vi "Ball Launcher Main.vi"() -> (4 "Elapsed Time":dbl, 15 "Error Out":errorcluster)   [LabVIEW 2023, in "Ball Launcher.lvlib"]
doc: "Sampe CLD Template"
uses:
  Ball Launcher.lvlib
  Typedefs/Queue Operations.ctl
  Typedefs/Data Cluster.ctl
  Typedefs/Timer Details.ctl
  <vilib>/Utility/error.llb/Trim Whitespace One-Sided.vi
panel:
  out "Ready":bool
  in  "Launch":bool
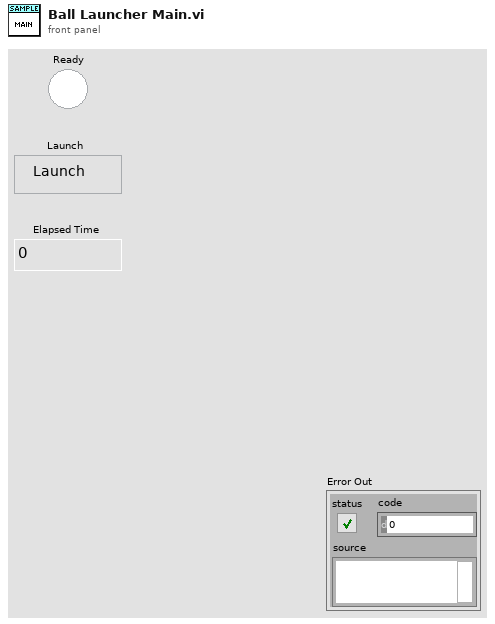
[diagram p1: front panel]
types:
  T1 = typedef "Ball Launcher.lvlib/Data Cluster.ctl" = cluster{"Timer Details":T2, "Enable Controls ref":refnum<vi>[], "Disable Controls ref":refnum<vi>[], "File Path":path, "Ready":bool}
  T2 = typedef "Ball Launcher.lvlib/Timer Details.ctl" = cluster{"Elapsed Time":dbl, "Previous Time":timestamp, "Started?":bool, "Set Time":dbl}
  T3 = typedef "Ball Launcher.lvlib/Queue Operations.ctl" = enum16{"Create Q", "Enqueue", "Enstack", "Dequeue", "Flush Q", "Release Q"}
  T4 = enum8{"Enabled", "Disabled", "Disabled and Grayed Out"}
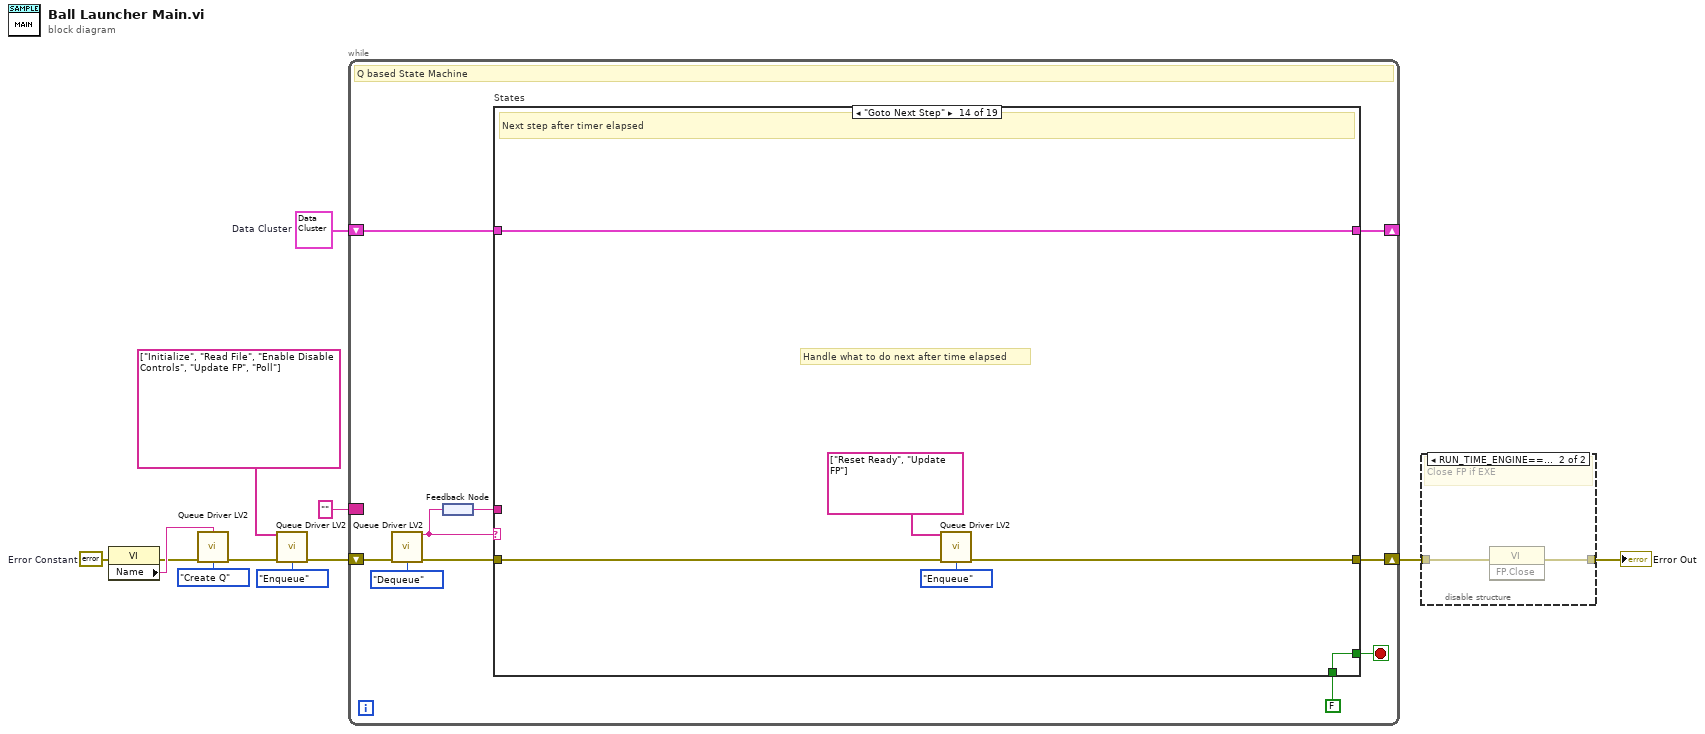
[diagram p0: block diagram]
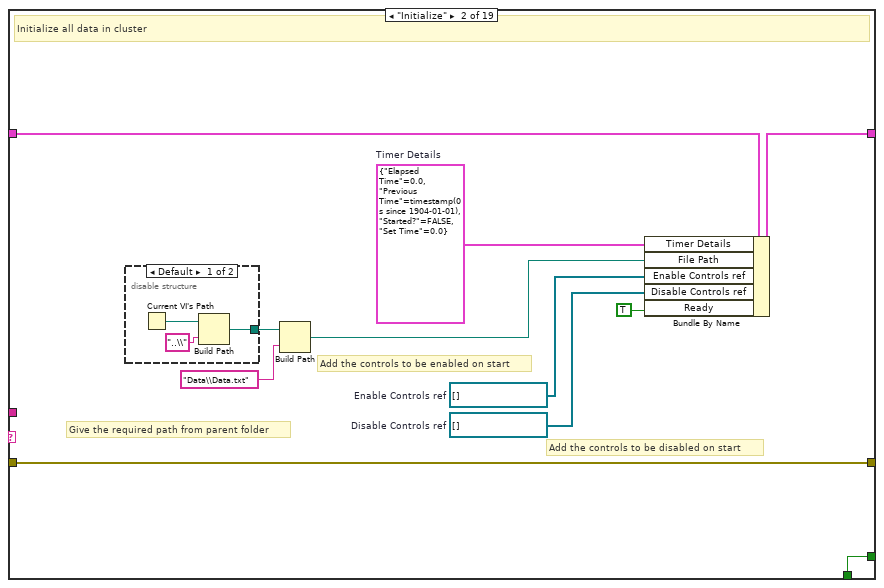
[diagram p4: hidden frame]
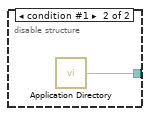
[diagram p5: hidden frame]
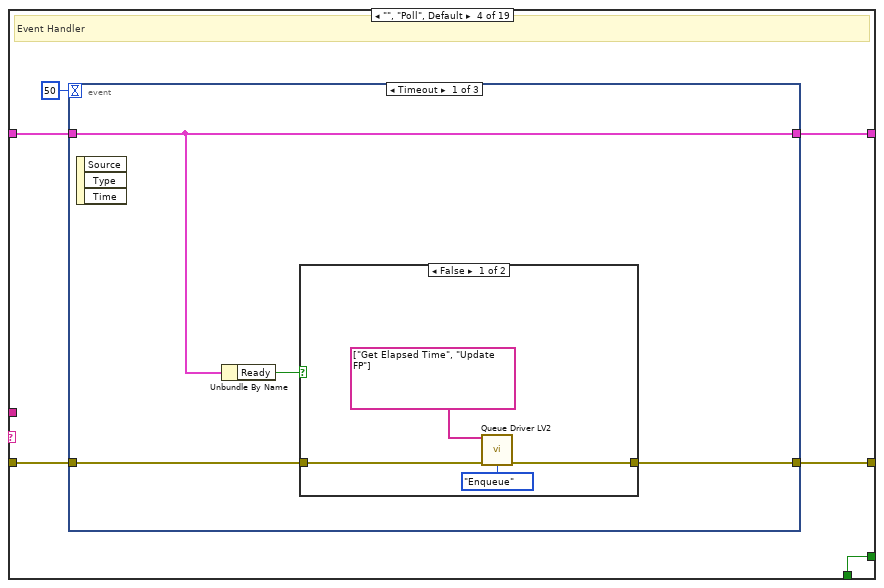
[diagram p7: hidden frame]
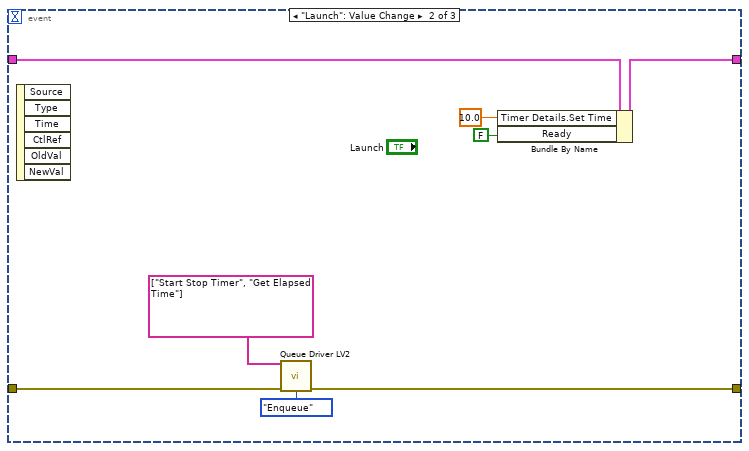
[diagram p9: hidden frame]
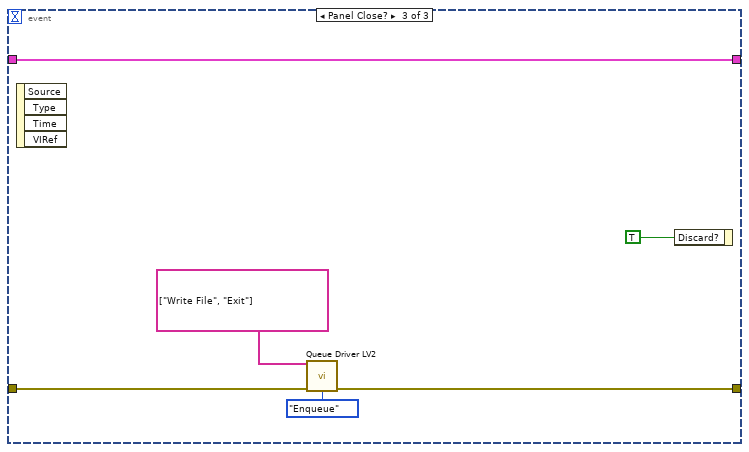
[diagram p10: hidden frame]
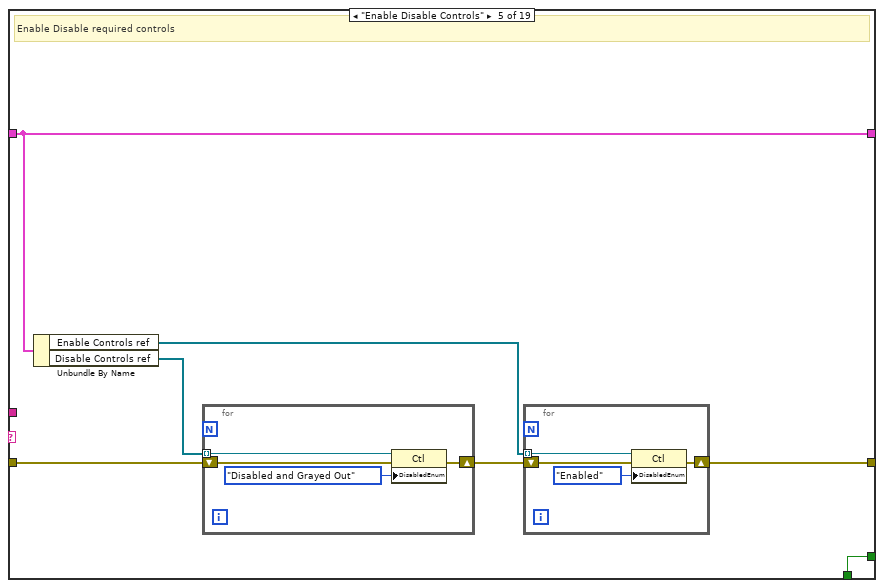
[diagram p11: hidden frame]
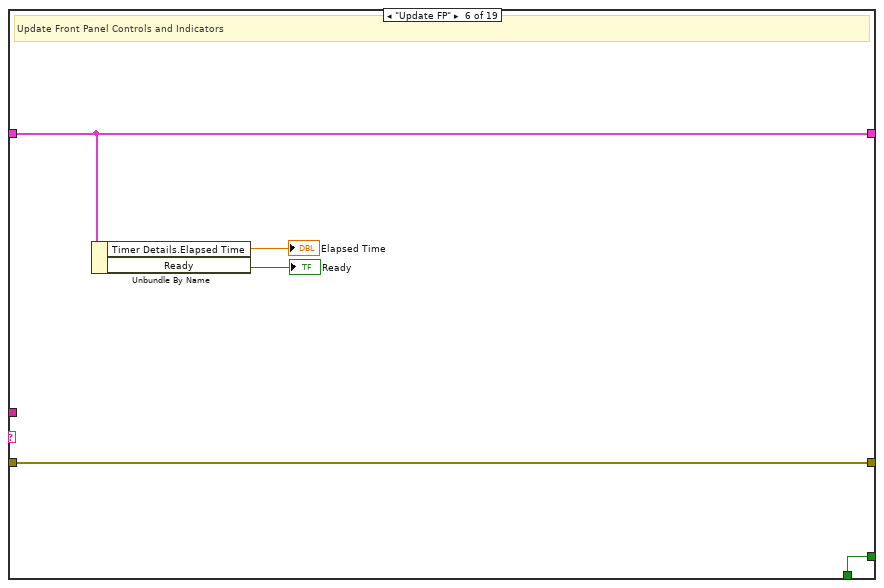
[diagram p12: hidden frame]
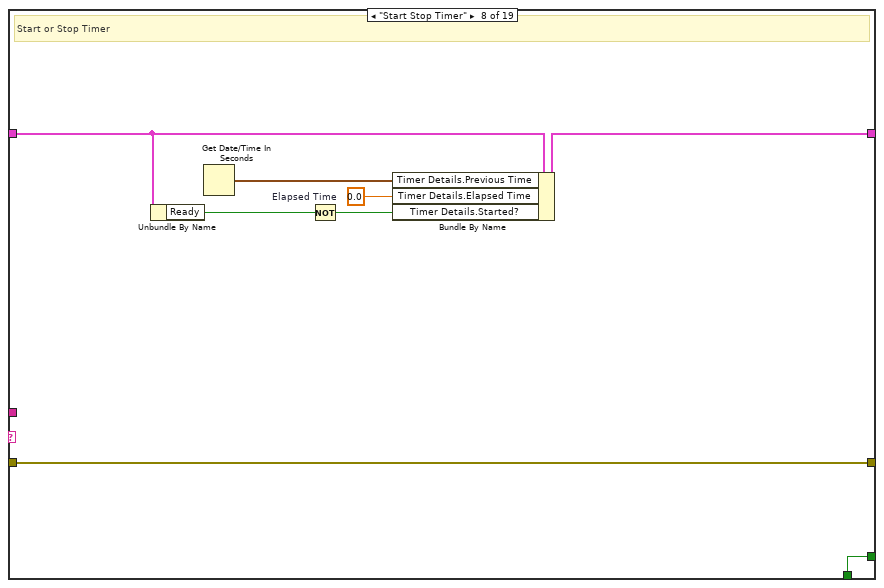
[diagram p14: hidden frame]
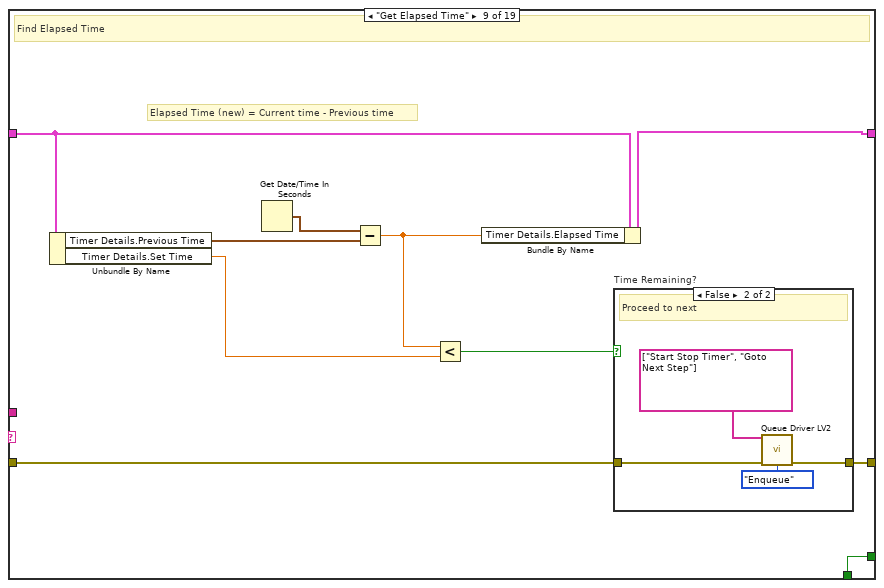
[diagram p15: hidden frame]
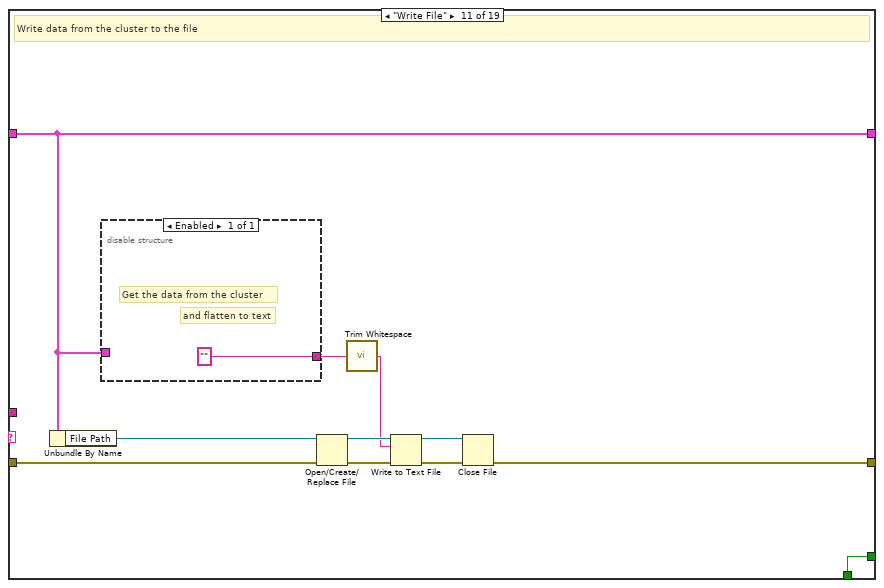
[diagram p18: hidden frame]
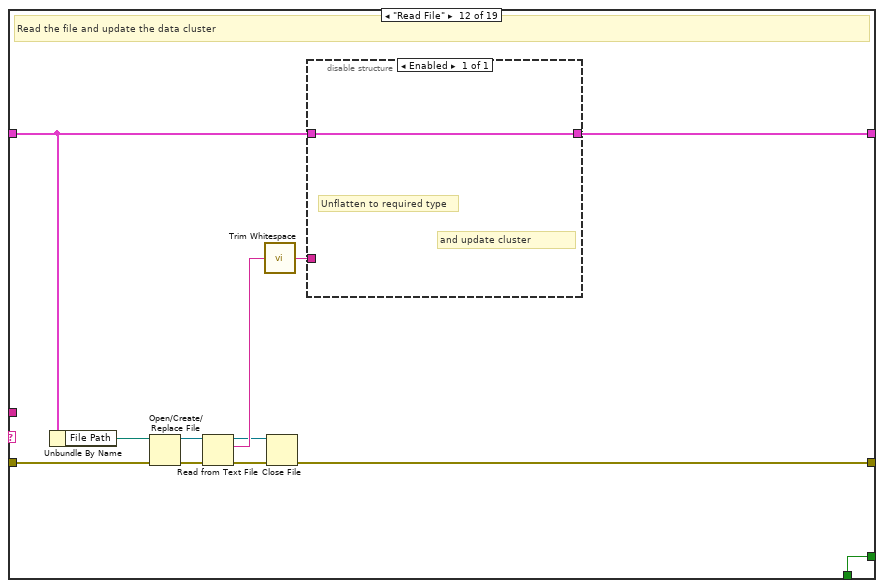
[diagram p19: hidden frame]
diagram:
  w1 = errorcluster {"status"=FALSE, "code"=0, "source"=""}  # Error Constant
  w4 = T1 {"Timer Details"={"Elapsed Time"=0.0, "Previous Time"=timestamp(0 s since 1904-01-01), "Started?"=FALSE, "Set Time"=0.0}, "Enable Controls ref"=[], "Disable Controls ref"=[], "File Path"=path "", "Ready"=FALSE}  # Data Cluster
  n1 = property class="VI"(error in=w1) -> (error out=w9:errorcluster, "Name"=w10:string)  [unwired: 1 in, 1 out]
  n2 = call "Queue Driver LV2.vi"("Name"=w10, "Error In"=w9, "Operation"=Queue_Operations."Create Q") -> ("error out"=w12:errorcluster)  [unwired: 11 in, 1 out]
  n3 = call "Queue Driver LV2.vi"("States[]"=string[] ["Initialize", "Read File", "Enable Disable Controls", "Update FP", "Poll"], "Error In"=w12, "Operation"=Queue_Operations."Enqueue") -> ("error out"=w11:errorcluster)  [unwired: 11 in, 1 out]
  n4 = while {
    border: "" ("States[]") -> [_]
    shift-right: [w17] -> w3
    shift-left: w11 -> [w22]
    shift-right: [w15] -> _
    shift-left: w4 -> [w16]
    stop <- w14 stop-if-true
    # "Q based State Machine"
    n5 = call "Queue Driver LV2.vi"("Error In"=w22, "Operation"=Queue_Operations."Dequeue") -> ("Dequeued State"=w19:string, "error out"=w21:errorcluster)  [unwired: 12 in]
    n6 = feedback-in #1(w19) -> ()
    n7 = feedback #1() -> (w18:string)
    n8 = case "States" shown="\"Goto Next Step\"" w19 {
      tunnel: w21 -> [w25 w36 w43 w49 w79 w92 w95 w103 w113 w121 w127 w144 w149 w151 w162 w165 w170 w189 w192]
      tunnel: w18 -> [_ _ _ _ _ _ _ _ _ _ _ _ _ _ _ _ w169 _ _]
      tunnel: [w25 w36 w43 w48 w75 w92 w95 w103 w106 w121 w125 w136 w149 w152 w162 w165 w166 w189 w191] -> w17
      tunnel: w16 -> [w24 w35 w42 w47 w74 w91 w94 w98 w108 w120 w123 w138 w148 w155 w159 w164 w179 w188 w196]
      tunnel: [w24 w34 w42 w46 w74 w91 w94 w102 w107 w120 w123 w137 w148 w155 w160 w164 w179 w188 w196] -> w15
      tunnel: FALSE -> [w23 w31 w41 w45 w73 w90 w93 w101 w105 w119 w132 w145 w147 w154 w161 w163 _ w187 _]
      tunnel: [w23 w31 w41 w45 w73 w90 w93 w101 w105 w119 w132 w145 w147 w154 w161 w163 TRUE w187 TRUE] -> w14
      frame "/***Initialize***/" {
      }
      frame "Initialize" {
        w32 = refnum<vi>[] []  # Disable Controls ref
        w33 = refnum<vi>[] []  # Enable Controls ref
        w27 = T2 {"Elapsed Time"=0.0, "Previous Time"=timestamp(0 s since 1904-01-01), "Started?"=FALSE, "Set Time"=0.0}  # Timer Details
        # "Give the required path from parent folder"
        # "Add the controls to be enabled on start"
        # "Add the controls to be disabled on start"
        # "Initialize all data in cluster"
        n9 = disable-structure shown="Default" {
          disable-tunnel: [w37 w40] -> w30
          frame condition #0 (active) {
            n10 = Current VI's Path() -> (path=w39:path)
            n11 = Build Path(base path=w39, name or relative path="..\\") -> (appended path=w37:path)
          }
          frame condition #1 {
            n12 = call <vilib>:"Application Directory.vi"() -> ("Application Directory"=w40:path)
          }
        }
        n13 = Build Path(base path=w30, name or relative path="Data\\Data.txt") -> (appended path=w28:path)
        n14 = Bundle By Name(cluster=w35, "Timer Details"=w27, "File Path"=w28, "Enable Controls ref"=w33, "Disable Controls ref"=w32, "Ready"=TRUE) -> (w34:T1)
      }
      frame "/***FP Related***/" {
      }
      frame "", "Poll", Default {
        # "Event Handler"
        n15 = event shown="[0] Timeout" {
          selector: _ -> [_ _ _]
          dyn-events: _ -> [_ _ _]
          timeout: 50 -> [_ _ _]
          tunnel: w49 -> [w53 w64 w68]
          tunnel: [w52 w65 w69] -> w48
          tunnel: w47 -> [w51 w61 w72]
          tunnel: [w51 w62 w72] -> w46
          event Timeout {
            n16 = event-data() -> ()  [unwired: 1 in, 3 out]
            n17 = Unbundle By Name(w51) -> ("Ready"=w50:bool)
            n18 = case shown="False" w50 {
              tunnel: w53 -> [w55 w58]
              tunnel: [w54 w58] -> w52
              frame False {
                n19 = call "Queue Driver LV2.vi"("States[]"=string[] ["Get Elapsed Time", "Update FP"], "Error In"=w55, "Operation"=Queue_Operations."Enqueue") -> ("error out"=w54:errorcluster)  [unwired: 11 in, 1 out]
              }
              frame True {
              }
            }
          }
          event "Launch": Value Change {
            n20 = event-data() -> ()  [unwired: 1 in, 6 out]
            n21 = call "Queue Driver LV2.vi"("States[]"=string[] ["Start Stop Timer", "Get Elapsed Time"], "Error In"=w64, "Operation"=Queue_Operations."Enqueue") -> ("error out"=w65:errorcluster)  [unwired: 11 in, 1 out]
            n22 = Bundle By Name(cluster=w61, "Timer Details.Set Time"=10.0, "Ready"=FALSE) -> (w62:T1)
          }
          event Panel Close? {
            n23 = event-data() -> ()  [unwired: 1 in, 4 out]
            n24 = call "Queue Driver LV2.vi"("States[]"=string[] ["Write File", "Exit"] ("Cases"), "Error In"=w68, "Operation"=Queue_Operations."Enqueue") -> ("error out"=w69:errorcluster)  [unwired: 11 in, 1 out]
            n25 = event-data("Discard?"=TRUE) -> ()  [unwired: 1 in, 1 out]
          }
        }
      }
      frame "Enable Disable Controls" {
        # "Enable Disable required controls"
        n26 = Unbundle By Name(w74) -> ("Enable Controls ref"=w76:refnum<vi>[], "Disable Controls ref"=w78:refnum<vi>[])
        n27 = for {
          shift-right: [w86] -> w77
          shift-left: w79 -> [w87]
          tunnel: w78 -> [w85] mode=indexing
          n28 = property class="Ctl"(reference=w85, error in=w87, "DisabledEnum"=T4."Disabled and Grayed Out" ("Disabled")) -> (error out=w86:errorcluster)  [unwired: 1 out]
        }
        n29 = for {
          shift-right: [w82] -> w75
          shift-left: w77 -> [w83]
          tunnel: w76 -> [w81] mode=indexing
          n30 = property class="Ctl"(reference=w81, error in=w83, "DisabledEnum"=T4."Enabled" ("Disabled")) -> (error out=w82:errorcluster)  [unwired: 1 out]
        }
      }
      frame "Update FP" {
        # "Update Front Panel Controls and Indicators"
        n31 = Unbundle By Name(w91) -> ("Timer Details.Elapsed Time"=→"Elapsed Time":dbl, "Ready"=→"Ready":bool)
      }
      frame "/***Timer Functions***/" {
      }
      frame "Start Stop Timer" {
        w100 = 0.0  # Elapsed Time
        # "Start or Stop Timer"
        n32 = Unbundle By Name(w98) -> ("Ready"=w97:bool)
        n33 = Get Date/Time In Seconds() -> (seconds since 1Jan1904=w99:timestamp)
        n34 = Not(x=w97) -> (.not. x?=w96:bool)
        n35 = Bundle By Name(cluster=w98, "Timer Details.Previous Time"=w99, "Timer Details.Elapsed Time"=w100, "Timer Details.Started?"=w96) -> (w102:T1)
      }
      frame "Get Elapsed Time" {
        # "Elapsed Time (new) = Current time - Previous time"
        # "Find Elapsed Time"
        n36 = Unbundle By Name(w108) -> ("Timer Details.Previous Time"=w112:timestamp, "Timer Details.Set Time"=w109:dbl)
        n37 = Get Date/Time In Seconds() -> (seconds since 1Jan1904=w111:timestamp)
        n38 = Subtract(x=w111, y=w112) -> (x-y=w110:dbl)
        n39 = Less?(x=w110, y=w109) -> (x < y?=w104:bool)
        n40 = Bundle By Name(cluster=w108, "Timer Details.Elapsed Time"=w110) -> (w107:T1)
        n41 = case "Time Remaining?" shown="False" w104 {
          tunnel: w113 -> [w114 w118]
          tunnel: [w114 w117] -> w106
          frame True {
            # "Continue"
          }
          frame False {
            # "Proceed to next"
            n42 = call "Queue Driver LV2.vi"("States[]"=string[] ["Start Stop Timer", "Goto Next Step"], "Error In"=w118, "Operation"=Queue_Operations."Enqueue") -> ("error out"=w117:errorcluster)  [unwired: 11 in, 1 out]
          }
        }
      }
      frame "/***File Operations***/" {
      }
      frame "Write File" {
        # "Write data from the cluster to the file"
        n43 = Unbundle By Name(w123) -> ("File Path"=w126:path)
        n44 = disable-structure shown="Enabled" {
          disable-tunnel: [""] -> w124
          disable-tunnel: w123 -> [_]
          frame Enabled {
            # "Get the data from the cluster"
            # "and flatten to text"
          }
        }
        n45 = Open/Create/Replace File(file path (use dialog)=w126, error in=w127) -> (refnum out=w128:refnum<file>, error out=w129:errorcluster)  [unwired: 4 in, 1 out]
        n46 = call <vilib>:"Trim Whitespace.vi"("string"=w124) -> ("trimmed string"=w122:string)  [unwired: 1 in]
        n47 = Write to Text File(file (use dialog)=w128, text=w122, error in=w129) -> (refnum out=w131:refnum<file>, error out=w130:errorcluster)  [unwired: 1 in, 1 out]
        n48 = Close File(refnum=w131, error in=w130) -> (error out=w125:errorcluster)  [unwired: 1 out]
      }
      frame "Read File" {
        # "Read the file and update the data cluster"
        n49 = Unbundle By Name(w138) -> ("File Path"=w140:path)
        n50 = Open/Create/Replace File(file path (use dialog)=w140, error in=w144) -> (refnum out=w141:refnum<file>, error out=w143:errorcluster)  [unwired: 4 in, 1 out]
        n51 = Read from Text File(file (use dialog)=w141, error in=w143) -> (refnum out=w135:refnum<file>, text=w139:string, error out=w142:errorcluster)  [unwired: 2 in, 1 out]
        n52 = call <vilib>:"Trim Whitespace.vi"("string"=w139) -> ("trimmed string"=w134:string)  [unwired: 1 in]
        n53 = Close File(refnum=w135, error in=w142) -> (error out=w136:errorcluster)  [unwired: 1 out]
        n54 = disable-structure shown="Enabled" {
          disable-tunnel: w134 -> [_]
          disable-tunnel: [w146] -> w137
          disable-tunnel: w138 -> [w146]
          frame Enabled {
            # "Unflatten to required type"
            # "and update cluster"
          }
        }
      }
      frame "/***Functionality***/" {
      }
      frame "Goto Next Step" {
        # "Handle what to do next after time elapsed"
        # "Next step after timer elapsed"
        n55 = call "Queue Driver LV2.vi"("States[]"=string[] ["Reset Ready", "Update FP"], "Error In"=w151, "Operation"=Queue_Operations."Enqueue") -> ("error out"=w152:errorcluster)  [unwired: 11 in, 1 out]
      }
      frame "Reset Ready" {
        n56 = Bundle By Name(cluster=w159, "Ready"=TRUE, "Timer Details.Elapsed Time"=0.0, "Timer Details.Started?"=FALSE) -> (w160:T1)
      }
      frame "/***Error***/" {
      }
      frame "Error" {
        # "Handle Errors"
        n57 = Unbundle By Name(w170) -> ("code"=w175:i32, "source"=w174:string)
        n58 = call <vilib>:"Clear Errors.vi"("error in (no error)"=w170, "specific error code to clear (0: all)"=w175) -> ("error out"=w177:errorcluster)  [unwired: 4 in, 1 out]
        n59 = Format Into String(format string="Error occurred in state \"%s\"!!\nError Code: %d\nError Source: %s\n\nDo you wish to continue?", error in=w177, w169, w175, w174) -> (resulting string=w173:string, error out=w167:errorcluster)  [unwired: 1 in]
        n60 = Two Button Dialog(message=w173, 1:"Exit" ("F button name (\"Cancel\")"), 2:"Continue" ("T button name (\"OK\")")) -> (T button?=w168:bool)
        n61 = case "Continue?" shown="False" w168 {
          tunnel: w167 -> [w184 w186]
          tunnel: [w180 w186] -> w166
          frame False {
            # "Exit"
            n62 = call "Queue Driver LV2.vi"("Error In"=w184, "Operation"=Queue_Operations."Flush Q") -> ("error out"=w181:errorcluster)  [unwired: 12 in, 1 out]
            n63 = call "Queue Driver LV2.vi"("States[]"=string[] ["Write File", "Initialize", "Enable Disable Controls", "Update FP", "Exit"], "Error In"=w181, "Operation"=Queue_Operations."Enqueue") -> ("error out"=w180:errorcluster)  [unwired: 11 in, 1 out]
          }
          frame True {
            # "Continue"
          }
        }
      }
      frame "/***Exit***/" {
      }
      frame "Exit" {
        # "Exit the State Machine"
        n64 = call "Queue Driver LV2.vi"("Error In"=w192, "Operation"=Queue_Operations."Flush Q") -> ("error out"=w195:errorcluster)  [unwired: 12 in, 1 out]
        n65 = call "Queue Driver LV2.vi"("Error In"=w195, "Operation"=Queue_Operations."Release Q") -> ("error out"=w191:errorcluster)  [unwired: 12 in, 1 out]
      }
    }
  }
  n66 = disable-structure shown="RUN_TIME_ENGINE==True" {
    disable-tunnel: w3 -> [w197 w199]
    disable-tunnel: [w197 w198] -> w2
    frame condition #0 (active) {
    }
    frame condition #1 {
      # "Close FP if EXE"
      n67 = invoke class="VI" method="FP.Close"(error in=w199) -> (error out=w198:errorcluster)  [unwired: 2 in, 2 out]
    }
  }
  "Error Out" <- w2
